vi "Calculate R assign_v1.vi"(8 "Assign Point":dbl[](array[numeric]), 9 "Eye Center":dbl[](array[numeric]), 10 "Rmax":dbl, 11 "Reye":dbl) -> (1 "Tassign":dbl[](array[numeric]), 3 "r_assign":dbl)   [LabVIEW 2010]
doc: "This VI calulates the assigned radius based on the formula:\nAssignPointRadius = min(EyeRadius - norm([ EyeCenter(1)-AssignPoint(1), EyeCenter(2)-AssignPoint(2) ],2),AssignPointRadiusMax)\n\nIf calculated AssignPointRadius is negative, namely the assign point is outside of the workspace, Rcalc would be 0 and Tcalc would be the starting point of the baseline trajectory."
uses:
  <vilib>/Analysis/NI_AALPro.lvlib
  <vilib>/Analysis/_algsub.llb/Real Vector Norm.vi
  <vilib>/Analysis/_algsub.llb/Vector Norm Type.ctl
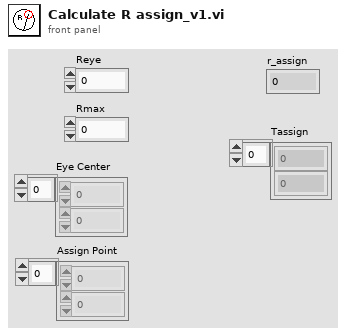
[diagram p1: front panel]
types:
  T1 = typedef "NI_AALPro.lvlib/Vector Norm Type.ctl" = u16
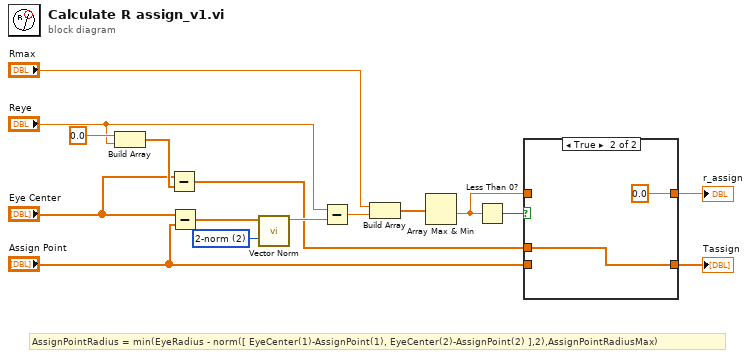
[diagram p0: block diagram]
diagram:
  w15 = T1 2 items=["1-norm"=1, "2-norm"=2, "Inf-norm"=3, "-Inf-norm"=4, "User Defined"=5] ("norm type")
  # "AssignPointRadius = min(EyeRadius - norm([ EyeCenter(1)-AssignPoint(1), EyeCenter(2)-AssignPoint(2) ],2),AssignPointRadiusMax)"
  n1 = Build Array(0.0 ("element"), "Reye") -> (w5:dbl[])
  n2 = Subtract(x="Eye Center", y=w5) -> (x-y=w3:dbl[])
  n3 = Subtract(x="Eye Center", y="Assign Point") -> (x-y=w16:dbl[])
  n4 = call-poly <vilib>:"Vector Norm.vi"("norm type"=w15, "Input Vector"=w16) -> ("norm"=w14:dbl)  [unwired: 8 in, 1 out]
  n5 = Subtract(x="Reye", y=w14) -> (x-y=w12:dbl)
  n6 = Build Array("Rmax", w12) -> (w11:dbl[])
  n7 = Array Max & Min(array=w11) -> (min value=w8:dbl)  [unwired: 3 out]
  n8 = Less Than 0?(x=w8) -> (x < 0?=w10:bool)
  n9 = case shown="True" w10 {
    tunnel: [w18 0.0] -> w9
    tunnel: w8 -> [w18 _]
    tunnel: "Assign Point" -> [w17 _]
    tunnel: [w17 w19] -> w6
    tunnel: w3 -> [_ w19]
    frame False {
    }
    frame True {
    }
  }
  "r_assign" <- w9
  "Tassign" <- w6
